vi "GUI_laptop v14.vi"() -> ()   [LabVIEW 2019]
uses:
  <vilib>/Math Plots/3D Math Plots/3D Scatter/3D Scatter XCtrl/3D Scatter.xctl
  <vilib>/Platform/TimedLoop/XDataNode/timing_clust.ctl
  <vilib>/Platform/TimedLoop/XDataNode/nitl_modes.ctl
  <vilib>/Platform/TimedLoop/XDataNode/wakeup.ctl
  <vilib>/Analysis/_algsub.llb/Real Vector Norm.vi
  <vilib>/Instr/_visa.llb/VISA Configure Serial Port (Instr).vi
  <vilib>/Utility/file.llb/Write Delimited Spreadsheet (DBL).vi
  <vilib>/addons/System Identification/Data Preprocess.llb/SI Lowpass Filter (MISO Array).vi
  <vilib>/Math Plots/3D Math Plots/3D Scatter/3D Scatter Datatype/Public/Plot Helper (Vector).vi
  <vilib>/platform/TimedLoop/XDataNode/XDataNode.xnode
  <vilib>/Platform/TimedLoop/XDataNode/XDNodeRunTimeDep.lvlib
  <vilib>/Analysis/NI_AALPro.lvlib
  <vilib>/Math Plots/3D Math Plots/3D Scatter/3D Scatter Datatype/3D Scatter Datatype.lvclass
  <vilib>/addons/System Identification/NI_SysID.lvlib
panel:
  out "Iteration Duration 2":i64
  out "Period":i64
  out "Actual End [i-1]":i64
  out "Expected End [i-1]":i64
  out "Finished Late? [i-1] 2":bool
  in  "Motion scale L3 outside rcm":dbl=2.0
  in  "L5 Deadzone":dbl
  in  "Sample rate":u32=200
  in  "Cutoff Frequency":dbl=10.0
  in  "Motion scale L1 L2":dbl=10.0
  in  "Motion scale L3":dbl=2.0
  in  "Save Path 4":path=path "C:/Users/jimmy/Documents/GitHub/Arduino-LabVIEW/zhantao/read_data_abs_filtered.csv"
  in  "Save Path 3":path=path "C:/Users/jimmy/Documents/GitHub/Arduino-LabVIEW/zhantao/read_data_abs_sending.csv"
  out "stimulus signals out":dbl[][](array[numeric]) format="%.2f"
  in  "L5 Offset":dbl
  in  "L5 Scale":dbl=1.0
  in  "Motion Scale L4":dbl=30.0
  out "spreadsheet string":string
  in  "Save Path 2":path=path "C:/Users/jimmy/Documents/GitHub/Arduino-LabVIEW/zhantao/read_data_delt.csv"
  out "send values":dbl[](array[numeric])
  out "Robot Feedback (l1 l2 l3 l4)":dbl[](array[numeric])
  in  "UDP Send":bool
  in  "UDP Recv":bool
  in  "L5 bound":dbl=1000.0
  in  "L4 bound (deg)":dbl=1000.0
  in  "L3 bound (mm)":dbl=1000.0
  in  "L2 bound (deg)":dbl=1000.0
  in  "L1 bound (deg)":dbl=1000.0
  in  "Joystick Type":dbl(ring)=1.0 items=["Rigid Joystick", "Free Joystick"]
  out "Finished Late? [i-1]":bool
  in  "Epsilon":dbl=0.2
  out "3D Scatter":refnum<class "3D Plot Datatype.lvclass">[](xcontrol)
  out "Random Point":dbl[](array[numeric])
  out "Virtual Cursor":dbl[](array[numeric])
  out "Iteration Duration":i64
  in  "Num of Points":i32=10
  in  "z bound":dbl=2.0
  in  "y bound":dbl=5.0
  in  "x bound":dbl=5.0
  in  "Stop":bool
  in  "Round Decimals":dbl=2.0 format="%#_15g"
  in  "Save Data":bool
  in  "Save Path":path=path "C:/Users/jimmy/Documents/GitHub/Arduino-LabVIEW/zhantao/read_data_abs.csv"
  in  "x speed":dbl=0.5
  in  "z speed":dbl=0.5
  in  "y speed":dbl=0.5
  out "error out":errorcluster
  in  "baud rate":u32=250000
  in  "VISA resource name":refnum<visa-resource-name>
  # "Joystick Selection"
  # "Plotting"
  # "Data Saving"
  # "Arduino Communication"
  # "Master Slave Communication"
  # "Parameters"
  # "TODO: add a lowpass filter for l5"
  # "TODO: fix the bounds; currently bounds are arbitrary"
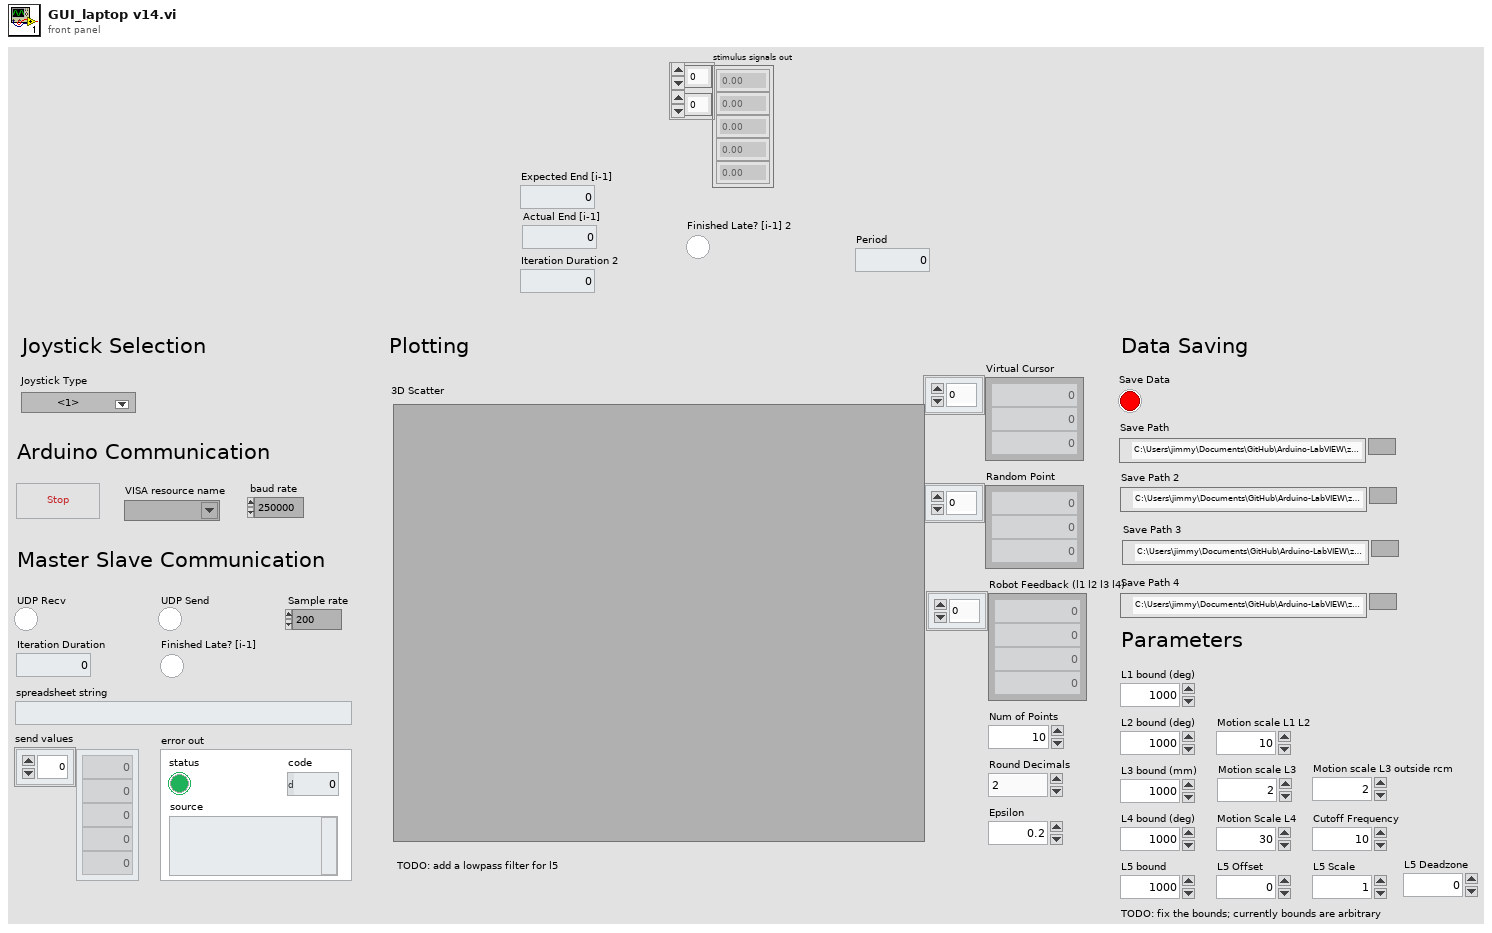
[diagram p1: front panel]
types:
  T1 = typedef "XDNodeRunTimeDep.lvlib/timing_clust.ctl" = cluster{"Expected End [f-1]":u64, "Actual End [f-1]":u64, "Finished Late? [f-1]":bool, "Expected End [i-1]":u64, "Actual End [i-1]":u64, "Finished Late? [i-1]":bool, "Expected Start [i]":u64, "Actual Start [i]":u64, "Expected Start [f]":u64, "Actual Start [f]":u64, "Source Name":string, "Structure Name":string, "Period":i64, "Deadline":i64, "Offset":i64, "Start":i64, "Priority":i32, "Timeout":i32, "Mode":T2, "Wakeup Reason":T3, "Error":errorcluster, "Source Type":string, "Secondary Source Type":string, "Global End Time":u64, "Global Start Time":u64, "Frame Duration":u64, "Iteration Duration":u64, "Assigned CPU":i32, "I/O Scan Engine Mode":u32}
  T2 = typedef "XDNodeRunTimeDep.lvlib/nitl_modes.ctl" = enum32{"No Change", "Process missed periods, maintain original phase", "Discard missed periods, maintain original phase", "Process missed periods, ignore original phase", "Discard missed periods, ignore original phase"}
  T3 = typedef "XDNodeRunTimeDep.lvlib/wakeup.ctl" = enum32{"Normal", "Aborted", "Asynchronous wakeup", "Timing source error", "Timed loop error", "Timeout"}
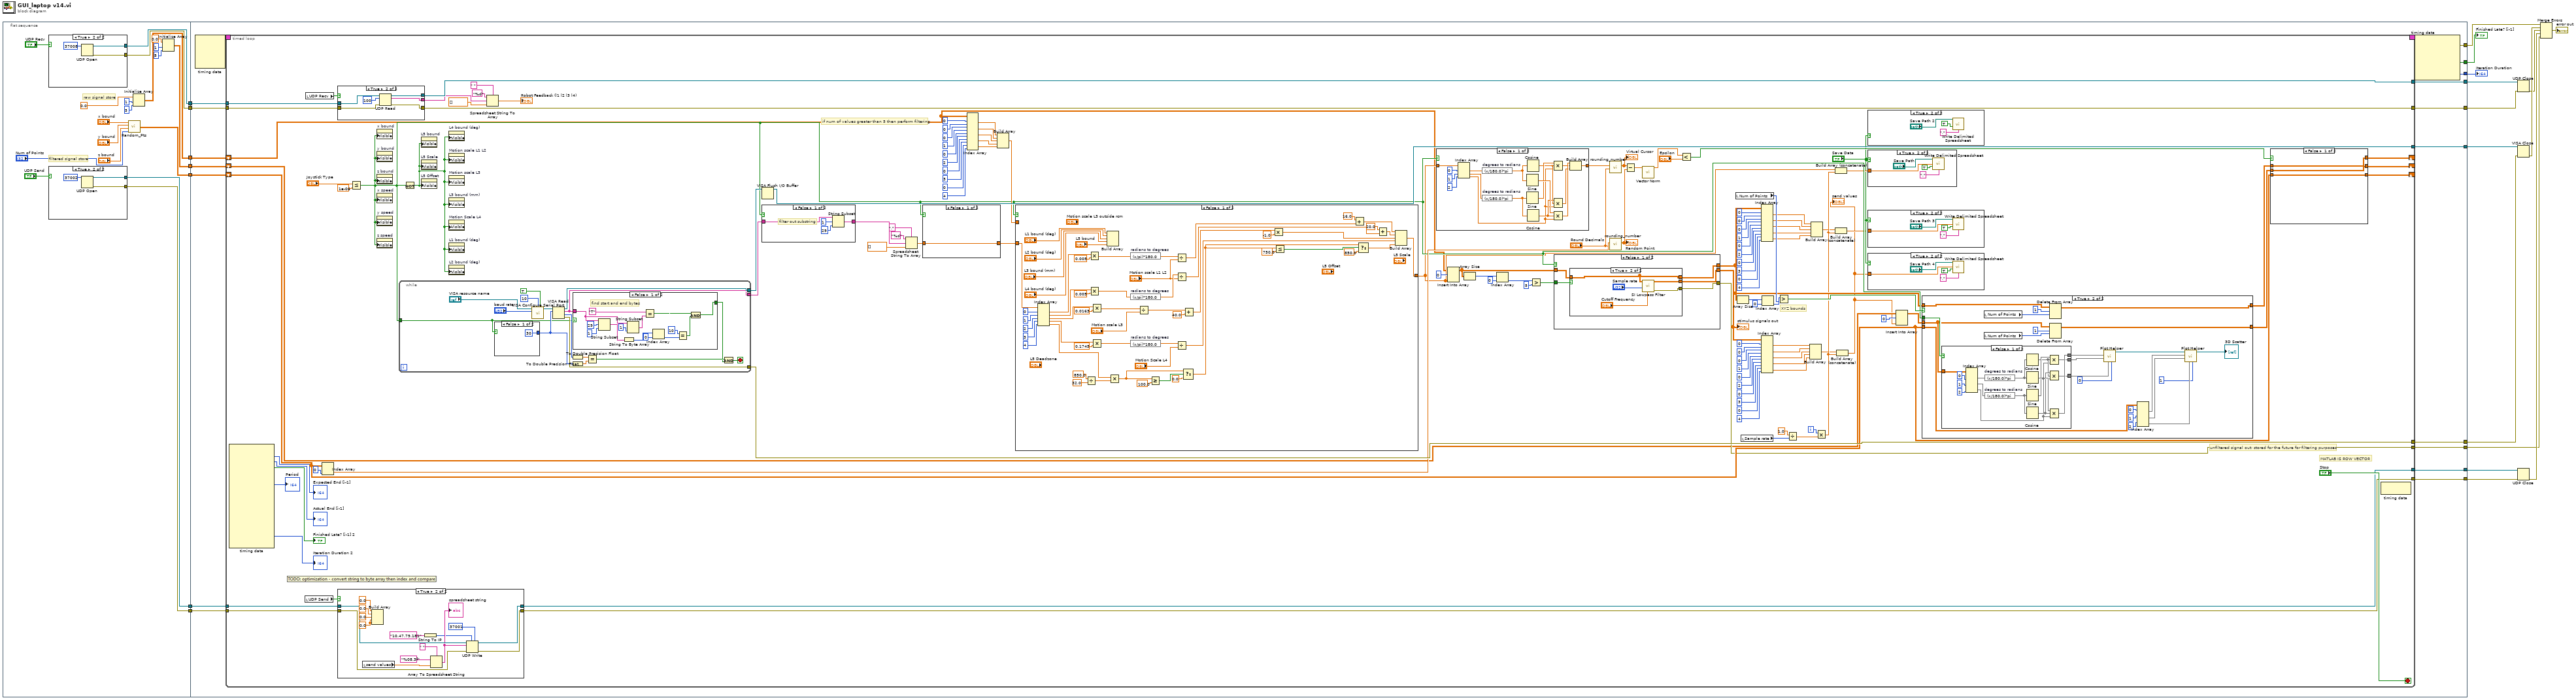
[diagram p0: block diagram]
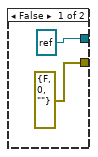
[diagram p2: hidden frame]
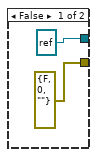
[diagram p3: hidden frame]
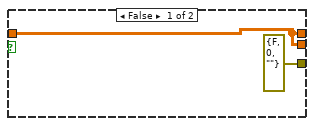
[diagram p6: hidden frame]
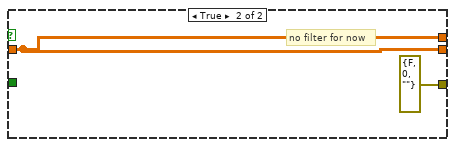
[diagram p7: hidden frame]
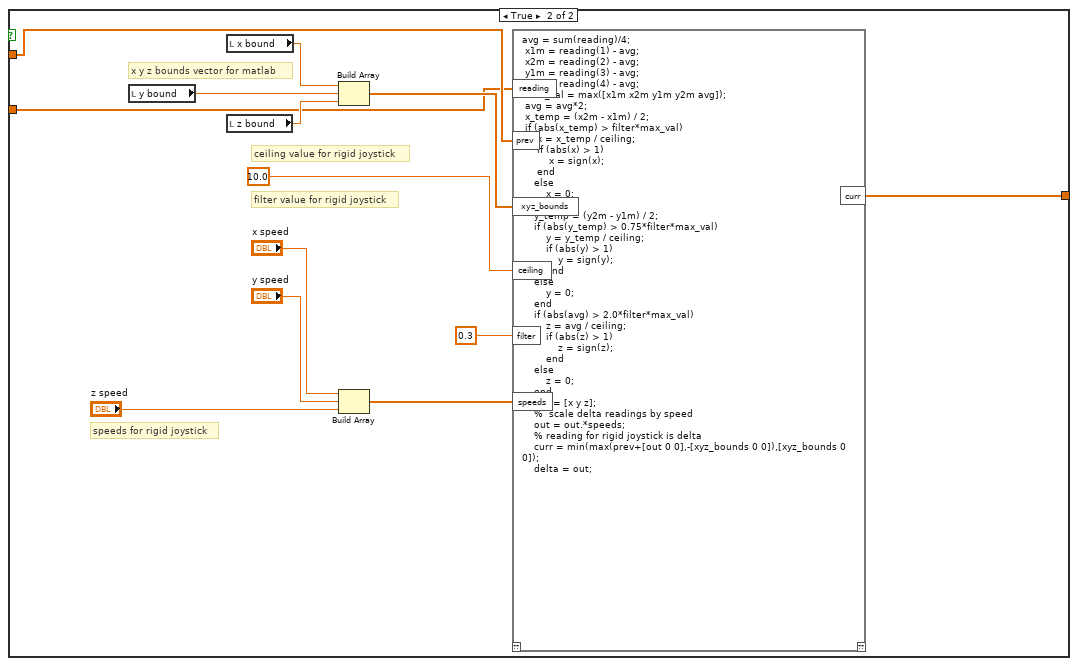
[diagram p8: hidden frame]
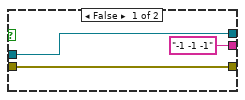
[diagram p11: hidden frame]
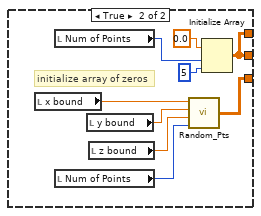
[diagram p13: hidden frame]
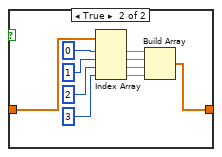
[diagram p15: hidden frame]
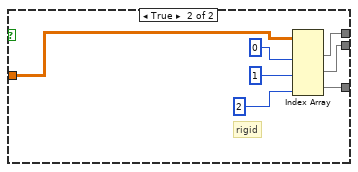
[diagram p18: hidden frame]
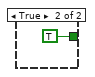
[diagram p19: hidden frame]
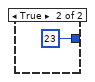
[diagram p20: hidden frame]
diagram:
  n1 = flat-sequence {
    tunnel: [w32] -> w18
    tunnel: [w36] -> w17
    tunnel: [w31] -> w16
    tunnel: [w30] -> w15
    tunnel: [w27] -> w14
    tunnel: [w26] -> w13
    tunnel: [w22] -> w2
    tunnel: [w67] -> w21
    tunnel: [w66] -> w20
    tunnel: [w64] -> w12
    tunnel: [w62] -> w19
    tunnel: w18 -> [w65]
    tunnel: w17 -> [w63]
    tunnel: w16 -> [w61]
    tunnel: w15 -> [w60]
    tunnel: w14 -> [w59]
    tunnel: w13 -> [w58]
    tunnel: [w57] -> w6
    tunnel: [w56] -> w11
    tunnel: [w55] -> w5
    tunnel: [w54] -> w4
    tunnel: [w53] -> w3
    tunnel: w2 -> [w52]
    tunnel: [w51] -> w1
    frame #0 {
      # "filtered signal store"
      # "raw signal store"
      n2 = case shown="True" "UDP Recv" {
        tunnel: [refnum<k16> refnum ("port") w49] -> w30
        tunnel: [errorcluster {"status"=FALSE, "code"=0, "source"=""} ("error out") w48] -> w27
        frame False {
        }
        frame True {
          n3 = UDP Open(11:u16 37008 ("port")) -> (port=w49:refnum<k16>, 0:w48:errorcluster)  [unwired: 4 in, 1 out]
        }
      }
      n4 = case shown="True" "UDP Send" {
        tunnel: [refnum<k16> refnum ("port") w44] -> w31
        tunnel: [errorcluster {"status"=FALSE, "code"=0, "source"=""} ("error out") w43] -> w26
        frame False {
        }
        frame True {
          n5 = UDP Open(11:u16 37002 ("port")) -> (port=w44:refnum<k16>, 0:w43:errorcluster)  [unwired: 4 in, 1 out]
        }
      }
      n6 = call "Random_Pts.vi"("Num of Points"="Num of Points", "z bound"="z bound", "y bound"="y bound", "x bound"="x bound") -> ("appended array"=w36:dbl[][])
      n7 = Initialize Array(0.0 ("element"), 1 ("dimension size"), 5 ("dimension size")) -> (w32:dbl[][])
      n8 = Initialize Array(0.0 ("element"), 1 ("dimension size"), 5 ("dimension size")) -> (w22:dbl[][])
    }
    frame #1 {
      n9 = node-c288() -> (w69:T1)  [unwired: 4 in]
      n10 = timed-loop {
        tunnel: [w140] -> w67
        tunnel: [w196] -> w66
        shift-right: [w195] -> _
        shift-left: w65 -> [w94]
        timing: w69 -> [_]
        timing-out: [_] -> w68
        shift-right: [w191] -> _
        shift-left: w63 -> [w192]
        tunnel: w61 -> [w154]
        tunnel: w60 -> [w153]
        tunnel: w59 -> [w151]
        tunnel: w58 -> [w150]
        tunnel: [w149] -> w57
        tunnel: [w148] -> w56
        tunnel: [w147] -> w55
        tunnel: [w146] -> w54
        tunnel: [w129] -> w53
        shift-right: [w86] -> _
        shift-left: w52 -> [w89]
        i -> [w84]
        stop <- "Stop" stop-if-true
        # "unfiltered signal out; stored for the future for filtering purposes"
        # "XYZ bounds"
        # "if num of values greater than 5 then perform filtering"
        # "MATLAB IS ROW VECTOR"
        n11 = node-c288() -> (→"Expected End [i-1]":i64, →"Actual End [i-1]":i64, →"Finished Late? [i-1] 2":bool, →"Period":i64, →"Iteration Duration 2":i64)  [unwired: 1 in, 12 out]
        n12 = local read "UDP Send"() -> (w79:bool)
        n13 = local read "UDP Recv"() -> (w152:bool)
        n14 = Index Array(array=w192, index (col)=0 ("index (row)")) -> (element=w163:dbl[])  [unwired: 1 in]
        n15 = case shown="True" w152 {
          tunnel: w153 -> [w309 w316]
          tunnel: w151 -> [w310 w315]
          tunnel: [w310 w314] -> w149
          tunnel: [w309 w313] -> w147
          tunnel: ["-1 -1 -1" w311] -> w142
          frame False {
          }
          frame True {
            n16 = UDP Read(connection ID=w316, max size (548)=100, 8:w315) -> (data out=w311:string, error out=w314:errorcluster, 3:w313:refnum<k16>)  [unwired: 1 in, 2 out]
          }
        }
        n17 = case shown="True" w79 {
          tunnel: w154 -> [w291 w307]
          tunnel: w150 -> [w292 w303]
          tunnel: [w292 w299] -> w148
          tunnel: [w291 w298] -> w146
          frame False {
          }
          frame True {
            w297 = 0.0 ("element")
            n18 = local read "send values"() -> (w293:dbl[])
            n19 = Build Array(0.0 ("element"), 0.0 ("element"), 0.0 ("element"), w297, w297) -> ()  [unwired: 1 out]
            n20 = String To IP(1:"10.47.79.181" ("name")) -> (0:w301:u32)
            n21 = Array To Spreadsheet String(delimiter (Tab)=" ", array=w293, 3:"%08.3f" ("format string")) -> (spreadsheet string=w304:string)
            "spreadsheet string" <- w304
            n22 = UDP Write(address=w301, port or service name=u16 37001, connection ID=w307, data in=w304, 8:w303) -> (error out=w299:errorcluster, 3:w298:refnum<k16>)  [unwired: 1 in]
          }
        }
        n23 = Less Or Equal?(x="Joystick Type", y=1e-06) -> (x <= y?=w130:bool)
        n24 = property on="x bound" class="DigNum (strict)"("Visible"=w130) -> ()  [unwired: 2 in, 2 out]
        n25 = property on="y bound" class="DigNum (strict)"("Visible"=w130) -> ()  [unwired: 2 in, 2 out]
        n26 = property on="z bound" class="DigNum (strict)"("Visible"=w130) -> ()  [unwired: 2 in, 2 out]
        n27 = property on="x speed" class="DigNum (strict)"("Visible"=w130) -> ()  [unwired: 2 in, 2 out]
        n28 = property on="y speed" class="DigNum (strict)"("Visible"=w130) -> ()  [unwired: 2 in, 2 out]
        n29 = property on="z speed" class="DigNum (strict)"("Visible"=w130) -> ()  [unwired: 2 in, 2 out]
        n30 = while {
          tunnel: [w415] -> w165
          tunnel: [w428] -> w196
          tunnel: [w422] -> w141
          tunnel: w130 -> [w416]
          stop <- w418 stop-if-true
          n31 = case shown="False" w416 {
            tunnel: [30 u32 23 ("byte count")] -> w421
            frame False {
            }
            frame True {
            }
          }
          n32 = call-poly "VISA Configure Serial Port"("VISA resource name"="VISA resource name", "termination char\n(0xA = '\\n' = LF)"=u8 10 ("termination char\n(0xA = '\\n' = LF)"), "Enable Termination\nChar (T)"=TRUE ("Enable Termination\nChar (T)"), "baud rate (9600)"="baud rate") -> ("VISA resource name out"=w423:refnum<visa-resource-name>)  [unwired: 10 in, 1 out]
          n33 = VISA Read(VISA resource name=w423, byte count=w421) -> (VISA resource name out=w422:refnum<visa-resource-name>, read buffer=w415:string, return count=w430:u32, error out=w428:errorcluster)  [unwired: 1 in]
          n34 = To Double Precision Float(number=w430) -> (double precision float=w429:dbl)
          n35 = To Double Precision Float(number=w421) -> (double precision float=w420:dbl)
          n36 = case shown="False" w416 {
            tunnel: [w437 TRUE] -> w417
            tunnel: w415 -> [w440 _]
            frame False {
              # "find start and end bytes"
              n37 = String Subset(string=w440, offset (0)=29, length (rest)=1) -> (substring=w435:string)
              n38 = String To Byte Array(string=w435) -> (unsigned byte array=w434:u8[])
              n39 = String Subset(string=w440, length (rest)=1) -> (substring=w443:string)  [unwired: 1 in]
              n40 = Equal?(x="T", y=w443) -> (x = y?=w439:bool)
              n41 = Index Array(array=w434, index=0) -> (element=w432:u8)
              n42 = Equal?(x=10, y=w432) -> (x = y?=w438:bool)
              n43 = And(x=w439, y=w438) -> (x .and. y?=w437:bool)
            }
            frame True {
            }
          }
          n44 = Equal?(x=w429, y=w420) -> (x = y?=w419:bool)
          n45 = And(x=w419, y=w417) -> (x .and. y?=w418:bool)
        }
        n46 = Not(x=w130) -> (.not. x?=w92:bool)
        n47 = property on="L5 bound" class="DigNum (strict)"("Visible"=w92) -> ()  [unwired: 2 in, 2 out]
        n48 = property on="L5 Scale" class="DigNum (strict)"("Visible"=w92) -> ()  [unwired: 2 in, 2 out]
        n49 = property on="L5 Offset" class="DigNum (strict)"("Visible"=w92) -> ()  [unwired: 2 in, 2 out]
        n50 = property on="L4 bound (deg)" class="DigNum (strict)"("Visible"=w92) -> ()  [unwired: 2 in, 2 out]
        n51 = property on="Motion scale L1 L2" class="DigNum (strict)"("Visible"=w92) -> ()  [unwired: 2 in, 2 out]
        n52 = property on="Motion scale L3" class="DigNum (strict)"("Visible"=w92) -> ()  [unwired: 2 in, 2 out]
        n53 = property on="L3 bound (mm)" class="DigNum (strict)"("Visible"=w92) -> ()  [unwired: 2 in, 2 out]
        n54 = property on="Motion Scale L4" class="DigNum (strict)"("Visible"=w92) -> ()  [unwired: 2 in, 2 out]
        n55 = property on="L1 bound (deg)" class="DigNum (strict)"("Visible"=w92) -> ()  [unwired: 2 in, 2 out]
        n56 = property on="L2 bound (deg)" class="DigNum (strict)"("Visible"=w92) -> ()  [unwired: 2 in, 2 out]
        n57 = Spreadsheet String To Array(delimiter (Tab)=" ", format string="%d", spreadsheet string=w142, array type (2D Dbl)=dbl[] []) -> (array=→"Robot Feedback (l1 l2 l3 l4)":dbl[])
        n58 = VISA Flush I/O Buffer(VISA resource name=w141) -> (VISA resource name out=w140:refnum<visa-resource-name>)  [unwired: 2 in, 1 out]
        n59 = case shown="False" w130 {
          tunnel: w165 -> [w336 w337]
          tunnel: [w333 w337] -> w164
          frame False {
            # "filter out substring"
            n60 = String Subset(string=w336, offset (0)=1, length (rest)=29) -> (substring=w333:string)
          }
          frame True {
          }
        }
        n61 = Spreadsheet String To Array(delimiter (Tab)=",", format string="%d", spreadsheet string=w164, array type (2D Dbl)=dbl[] []) -> (array=w166:dbl[])
        n62 = case shown="False" w130 {
          tunnel: w166 -> [w338 w342]
          tunnel: [w338 w341] -> w138
          frame False {
          }
          frame True {
            n63 = Index Array(array=w342, index #1=0 ("Plot ID"), index #2=1 ("Plot ID"), index #3=2 ("Plot ID"), index #4=3 ("index")) -> (element #1=w345:dbl, element #2=w344:dbl, element #3=w343:dbl, element #4=w339:dbl)
            n64 = Build Array(w345, w344, w343, w339) -> (w341:dbl[])
          }
        }
        n65 = Index Array(array=w94, index (row) #1=0 ("disabled index (row)"), index (col) #1=0 ("disabled index (col)"), index (row) #2=0 ("disabled index (row)"), index (col) #2=1 ("disabled index (col)"), index (row) #3=0 ("disabled index (row)"), index (col) #3=2 ("disabled index (col)"), index (row) #4=0 ("disabled index (row)"), index (col) #4=3 ("disabled index (col)"), index (row) #5=0 ("disabled index (row)"), index (col) #5=4 ("disabled index (col)")) -> (element #1=w177:dbl, element #2=w176:dbl, element #3=w175:dbl, element #4=w168:dbl, element #5=w167:dbl)
        n66 = Build Array(w177, w176, w175, w168, w167) -> (w139:dbl[])
        n67 = case shown="False" w130 {
          tunnel: w139 -> [_ w277]
          tunnel: w138 -> [w264 w276]
          tunnel: [w225 w275] -> w113
          frame False {
            n68 = Index Array(array=w264, index #1=0 ("Plot ID"), index #2=1 ("Plot ID"), index #3=2 ("Plot ID"), index #4=3 ("Plot ID"), index #5=4 ("Plot ID")) -> (element #1=w263:dbl, element #2=w251:dbl, element #3=w243:dbl, element #4=w241:dbl, element #5=w224:dbl)
            n69 = Divide(x=850.0, y=32.0) -> (x/y=w221:dbl)
            n70 = Multiply(x=w263, y=0.005) -> (x*y=w259:dbl)
            n71 = Multiply(x=w251, y=0.005) -> (x*y=w254:dbl)
            n72 = Multiply(x=w243, y=0.0163) -> (x*y=w247:dbl)
            n73 = Multiply(x=w241, y=0.1745) -> (x*y=w240:dbl)
            n74 = Build Array("L1 bound (deg)", "L2 bound (deg)", "L3 bound (mm)", "L4 bound (deg)", "L5 bound") -> ()  [unwired: 1 out]
            n75 = Multiply(x=w224, y=w221) -> (x*y=w220:dbl)
            n76 = expression code="(x/pi)*180.0" "radians to degrees"(w259) -> (w258:dbl)
            n77 = expression code="(x/pi)*180.0" "radians to degrees"(w254) -> (w253:dbl)
            n78 = expression code="(x/pi)*180.0" "radians to degrees"(w240) -> (w239:dbl)
            n79 = Divide(x=w247, y="Motion scale L3") -> (x/y=w245:dbl)
            n80 = Greater Or Equal?(x=w220, y=100.0) -> (x >= y?=w232:bool)
            n81 = Divide(x=w258, y="Motion scale L1 L2") -> (x/y=w261:dbl)
            n82 = Divide(x=w253, y="Motion scale L1 L2") -> (x/y=w256:dbl)
            n83 = Divide(x=w239, y="Motion Scale L4") -> (x/y=w234:dbl)
            n84 = Select(t=w220, s=w232, f=0.0) -> (s? t:f=w227:dbl)
            n85 = Add(x=w245, y=40.0) -> (x+y=w249:dbl)
            n86 = Multiply(x=w249, y=-1.0) -> (x*y=w235:dbl)
            n87 = Less Or Equal?(x=w227, y=750.0) -> (x <= y?=w228:bool)
            n88 = Add(x=16.0, y=w261) -> (x+y=w237:dbl)
            n89 = Select(t=w227, s=w228, f=850.0) -> (s? t:f=w226:dbl)
            n90 = Add(x=20.0, y=w256) -> (x+y=w236:dbl)
            n91 = Build Array(w237, w236, w235, w234, w226) -> (w225:dbl[])
          }
          frame True {
            # "ceiling value for rigid joystick"
            # "filter value for rigid joystick"
            # "speeds for rigid joystick"
            # "x y z bounds vector for matlab"
            n92 = local read "y bound"() -> (w286:dbl)
            n93 = local read "x bound"() -> (w285:dbl)
            n94 = local read "z bound"() -> (w287:dbl)
            n95 = Build Array(w285, w286, w287) -> (w278:dbl[])
            n96 = Build Array("x speed", "y speed", "z speed") -> (w281:dbl[])
            n97 = script code="avg = sum(reading)/4;\n x1m = reading(1) - avg;\n x2m = reading(2) - avg;\n y1m = reading(3) - avg;\n y2m = reading(4) - avg;\n max_val = max([x1m x2m y1m y2m avg]);\n avg = avg*2;\n x_temp = (x2m - x1m) / 2;\n if (abs(x_temp) > filter*max_val)\n     x = x_temp / ceiling;\n     if (abs(x) > 1)\n         x = sign(x);\n     end\n    else\n        x = 0;\n    end\n    y_temp = (y2m - y1m) / 2;\n    if (abs(y_temp) > 0.75*filter*max_val)\n        y = y_temp / ceiling;\n        if (abs(y) > 1)\n            y = sign(y);\n        end\n    else\n        y = 0;\n    end\n    if (abs(avg) > 2.0*filter*max_val)\n        z = avg / ceiling;\n        if (abs(z) > 1)\n            z = sign(z);\n        end\n    else\n        z = 0;\n    end\n    out = [x y z];\n    %  scale delta readings by speed\n    out = out.*speeds;\n    % reading for rigid joystick is delta\n    curr = min(max(prev+[out 0 0],-[xyz_bounds 0 0]),[xyz_bounds 0 0]);\n    delta = out;"("xyz_bounds"=w278, "ceiling"=10.0 ("Real"), "filter"=0.3 ("Real"), "speeds"=w281, "reading"=w276, "prev"=w277) -> ("curr"=w275:dbl[])  [unwired: 1 in, 1 out]
          }
        }
        n98 = case shown="False" w130 {
          tunnel: [w362 w366] -> w193
          tunnel: w113 -> [w361 w366]
          frame False {
            n99 = Index Array(array=w361, index #1=0 ("Plot ID"), index #2=1 ("Plot ID"), index #3=2 ("Plot ID")) -> (element #1=w360:dbl, element #2=w359:dbl, element #3=w349:dbl)
            n100 = expression code="(x/180.0)*pi" "degrees to radians"(w360) -> (w358:dbl)
            n101 = expression code="(x/180.0)*pi" "degrees to radians"(w359) -> (w357:dbl)
            n102 = Sine(x=w358) -> (sin(x)=w355:dbl)
            n103 = Sine(x=w357) -> (sin(x)=w354:dbl)
            n104 = Cosine(x=w358) -> (cos(x)=w351:dbl)
            n105 = Cosine(x=w357) -> (cos(x)=w352:dbl)
            n106 = Compound Arithmetic op=MULTIPLY(w354, w351, w349) -> (w353:dbl)
            n107 = Compound Arithmetic op=MULTIPLY(w352, w351, w349) -> (w350:dbl)
            n108 = Compound Arithmetic op=MULTIPLY(w355, w352, w349) -> (w356:dbl)
            n109 = Build Array(w356, w353, w350) -> (w362:dbl[])
          }
          frame True {
          }
        }
        n110 = Insert Into Array(array=w94, index (row)=0, new element=w113) -> (w131:dbl[][])  [unwired: 1 in]
        n111 = Array Size(array=w131) -> (size(s)=w134:i32[])
        n112 = Index Array(array=w134, index=0) -> (element=w133:i32)
        n113 = Greater?(x=w133, y=5) -> (0:w80:bool)
        n114 = case shown="False" w130 {
          tunnel: w80 -> [w208 _]
          tunnel: w131 -> [w210 w218]
          tunnel: [w209 w218] -> w91
          tunnel: [w207 errorcluster {"status"=FALSE, "code"=0, "source"=""} ("error out")] -> w129
          tunnel: [w206 w218] -> w95
          frame False {
            n115 = case shown="True" w208 {
              tunnel: w210 -> [w211 w216]
              tunnel: [w211 w216] -> w209
              tunnel: [errorcluster {"status"=FALSE, "code"=0, "source"=""} ("error out") w217] -> w207
              tunnel: [w211 w215] -> w206
              frame False {
              }
              frame True {
                n116 = call-poly <vilib>:"SI Lowpass Filter.vi"("cutoff frequency"="Cutoff Frequency", "sampling rate (Hz)"="Sample rate", "stimulus signals in"=w216) -> ("error out"=w217:errorcluster, "stimulus signals out"=w215:dbl[][])  [unwired: 6 in, 1 out]
              }
            }
          }
          frame True {
            # "no filter for now"
          }
        }
        "stimulus signals out" <- w95
        n117 = call "rounding_number.vi"("power of ten"="Round Decimals", "Array"=w193) -> ("rounded"=w161:dbl[])  [unwired: 9 in]
        "Virtual Cursor" <- w161
        n118 = call "rounding_number.vi"("power of ten"="Round Decimals", "Array"=w163) -> ("rounded"=w160:dbl[])  [unwired: 9 in]
        "Random Point" <- w160
        n119 = Subtract(x=w161, y=w160) -> (x-y=w159:dbl[])
        n120 = call-poly <vilib>:"Vector Norm.vi"("Input Vector"=w159) -> ("norm"=w158:dbl)  [unwired: 9 in, 1 out]
        n121 = Less?(x=w158, y="Epsilon") -> (x < y?=w156:bool)
        n122 = local read "Num of Points"() -> (w179:i32)
        n123 = Array Size(array=w91) -> (size(s)=w137:i32[])
        n124 = local read "Sample rate"() -> (w81:u32)
        n125 = Index Array(array=w91, index (row) #1=0 ("disabled index (col)"), index (col) #1=0 ("disabled index (row)"), index (row) #2=0 ("disabled index (col)"), index (col) #2=1 ("disabled index (row)"), index (row) #3=0 ("disabled index (col)"), index (col) #3=2 ("disabled index (row)"), index (row) #4=0 ("disabled index (col)"), index (col) #4=3 ("disabled index (row)"), index (row) #5=0 ("disabled index (col)"), index (col) #5=4 ("disabled index (col)")) -> (element #1=w118:dbl, element #2=w117:dbl, element #3=w116:dbl, element #4=w115:dbl, element #5=w114:dbl)
        n126 = Index Array(array=w95, index (row) #1=0 ("disabled index (col)"), index (col) #1=0 ("disabled index (row)"), index (row) #2=0 ("disabled index (col)"), index (col) #2=1 ("disabled index (row)"), index (row) #3=0 ("disabled index (col)"), index (col) #3=2 ("disabled index (row)"), index (row) #4=0 ("disabled index (col)"), index (col) #4=3 ("disabled index (row)"), index (row) #5=0 ("disabled index (col)"), index (col) #5=4 ("disabled index (col)")) -> (element #1=w101:dbl, element #2=w100:dbl, element #3=w99:dbl, element #4=w98:dbl, element #5=w97:dbl)
        n127 = Index Array(array=w137, index=0) -> (element=w180:i32)
        n128 = Greater?(x=w180, y=w179) -> (0:w178:bool)
        n129 = Divide(x=1.0, y=w81) -> (x/y=w82:dbl)
        n130 = Build Array(w101, w100, w99, w98, w97) -> (w78:dbl[])
        n131 = Build Array(w118, w117, w116, w115, w114) -> (w77:dbl[])
        n132 = Multiply(x=w84, y=w82) -> (x*y=w85:dbl)
        n133 = Build Array (concatenate)(w113, w85) -> (w112:dbl[])
        n134 = Build Array (concatenate)(w77, w85) -> (w93:dbl[])
        n135 = Build Array (concatenate)(w78, w85) -> (w70:dbl[])
        "send values" <- w70
        n136 = case shown="True" "Save Data" {
          frame False {
          }
          frame True {
            n137 = call-poly <vilib>:"Write Delimited Spreadsheet.vi"("file path (dialog if empty)"="Save Path 2", "append to file? (new file:F)"=TRUE, "delimiter (\\t)"="," ("delimiter (\\t)")) -> ()  [unwired: 11 in, 2 out]
          }
        }
        n138 = case shown="True" "Save Data" {
          tunnel: w112 -> [_ w317]
          frame False {
          }
          frame True {
            n139 = call-poly <vilib>:"Write Delimited Spreadsheet.vi"("file path (dialog if empty)"="Save Path", "1D data"=w317, "append to file? (new file:F)"=TRUE, "delimiter (\\t)"="," ("delimiter (\\t)")) -> ()  [unwired: 10 in, 2 out]
          }
        }
        n140 = case shown="True" "Save Data" {
          tunnel: w93 -> [_ w202]
          frame False {
          }
          frame True {
            n141 = call-poly <vilib>:"Write Delimited Spreadsheet.vi"("file path (dialog if empty)"="Save Path 3", "1D data"=w202, "append to file? (new file:F)"=TRUE, "delimiter (\\t)"="," ("delimiter (\\t)")) -> ()  [unwired: 10 in, 2 out]
          }
        }
        n142 = case shown="True" "Save Data" {
          tunnel: w70 -> [_ w198]
          frame False {
          }
          frame True {
            n143 = call-poly <vilib>:"Write Delimited Spreadsheet.vi"("file path (dialog if empty)"="Save Path 4", "1D data"=w198, "append to file? (new file:F)"=TRUE, "delimiter (\\t)"="," ("delimiter (\\t)")) -> ()  [unwired: 10 in, 2 out]
          }
        }
        n144 = Insert Into Array(array=w89, index (row)=0, new element=w70) -> (w88:dbl[][])  [unwired: 1 in]
        n145 = case shown="True" w178 {
          tunnel: w91 -> [w368 w390]
          tunnel: [w368 w389] -> w194
          tunnel: w192 -> [w367 w388]
          tunnel: w130 -> [_ w373]
          tunnel: w88 -> [_ w370]
          tunnel: [w367 w369] -> w87
          frame False {
          }
          frame True {
            n146 = case shown="False" w373 {
              tunnel: w370 -> [w407 w411]
              tunnel: [w394 w410] -> w379
              tunnel: [w393 w409] -> w378
              tunnel: [w392 w408] -> w377
              frame False {
                n147 = Index Array(array=w407, index (col) #1=0 ("Plot ID"), index (col) #2=1 ("Plot ID"), index (col) #3=2 ("Plot ID")) -> (element #1=w397:dbl[], element #2=w396:dbl[], element #3=w395:dbl[])  [unwired: 3 in]
                n148 = expression code="(x/180.0)*pi" "degrees to radians"(w397) -> (w403:dbl[])
                n149 = expression code="(x/180.0)*pi" "degrees to radians"(w396) -> (w402:dbl[])
                n150 = Cosine(x=w403) -> (cos(x)=w398:dbl[])
                n151 = Sine(x=w403) -> (sin(x)=w401:dbl[])
                n152 = Sine(x=w402) -> (sin(x)=w400:dbl[])
                n153 = Cosine(x=w402) -> (cos(x)=w399:dbl[])
                n154 = Compound Arithmetic op=MULTIPLY(w400, w398, w395) -> (w393:dbl[])
                n155 = Compound Arithmetic op=MULTIPLY(w399, w398, w395) -> (w392:dbl[])
                n156 = Compound Arithmetic op=MULTIPLY(w401, w399, w395) -> (w394:dbl[])
              }
              frame True {
                # "rigid"
                n157 = Index Array(array=w411, index (col) #1=0 ("disabled index (col)"), index (col) #2=1 ("index (col)"), index (col) #3=2 ("index (col)")) -> (element #1=w410:dbl[], element #2=w409:dbl[], element #3=w408:dbl[])  [unwired: 3 in]
              }
            }
            n158 = local read "Num of Points"() -> (w387:i32)
            n159 = local read "Num of Points"() -> (w372:i32)
            n160 = Delete From Array(array=w390, length=1, index (row)=w387) -> (array with subset deleted=w389:dbl[][])  [unwired: 1 in, 1 out]
            n161 = Delete From Array(array=w370, length=1, index (row)=w372) -> (array with subset deleted=w369:dbl[][])  [unwired: 1 in, 1 out]
            n162 = call-poly <vilib>:"Plot Helper.vi"("Plot ID"=0, "z vector"=w377, "y vector"=w378, "x vector"=w379) -> ("3D Plot lvclass Array out"=w381:refnum<class "3D Plot Datatype.lvclass">[])  [unwired: 2 in, 5 out]
            n163 = Index Array(array=w388, index (row) #1=0 ("index (row)"), index (row) #2=1 ("index (row)"), index (row) #3=2 ("index (row)")) -> (element #1=w385:dbl[], element #2=w384:dbl[], element #3=w383:dbl[])  [unwired: 3 in]
            n164 = call-poly <vilib>:"Plot Helper.vi"("Plot ID"=1, "z vector"=w383, "y vector"=w384, "x vector"=w385, "3D Plot lvclass Array in"=w381) -> ("3D Plot lvclass Array out"=→"3D Scatter":refnum<class "3D Plot Datatype.lvclass">[])  [unwired: 1 in, 5 out]
          }
        }
        n165 = case shown="False" w156 {
          tunnel: w192 -> [w323 _]
          tunnel: [w323 w328] -> w191
          tunnel: w194 -> [w322 _]
          tunnel: [w322 w324] -> w195
          tunnel: w87 -> [w321 _]
          tunnel: [w321 w324] -> w86
          frame False {
          }
          frame True {
            # "initialize array of zeros"
            n166 = local read "x bound"() -> (w332:dbl)
            n167 = local read "Num of Points"() -> (w326:i32)
            n168 = local read "Num of Points"() -> (w329:i32)
            n169 = local read "y bound"() -> (w331:dbl)
            n170 = local read "z bound"() -> (w330:dbl)
            n171 = call "Random_Pts.vi"("Num of Points"=w329, "z bound"=w330, "y bound"=w331, "x bound"=w332) -> ("appended array"=w328:dbl[][])
            n172 = Initialize Array(0.0 ("element"), w326, 5 ("dimension size")) -> (w324:dbl[][])
          }
        }
        n173 = node-c288() -> ()  [unwired: 1 in, 1 out]
      }
      n174 = node-c288(w68) -> (w64:errorcluster, w51:bool, w62:i64)  [unwired: 3 out]
    }
  }
  n175 = UDP Close(connection ID=w5, 8:w6) -> (error out=w9:errorcluster)  [unwired: 1 out]
  n176 = VISA Close(VISA resource name=w21, error in (no error)=w20) -> (error out=w10:errorcluster)
  n177 = UDP Close(connection ID=w4, 8:w11) -> (error out=w8:errorcluster)  [unwired: 1 out]
  n178 = Merge Errors(w12, w10, w9, w8, w3) -> (→"error out":errorcluster)
  "Iteration Duration" <- w19
  "Finished Late? [i-1]" <- w1
